vi "Configure Trigger.vi"   [LabVIEW 2015, in "LeCroy Wave Series.lvlib"]
doc: "This VI select the type of trigger."
uses:
  <instrlib>/LeCroy Wave Series/LeCroy Wave Series.lvlib
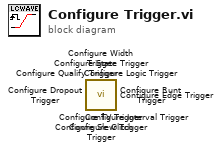
[diagram p0: block diagram]
diagram:
  n1 = call <instrlib>:"Configure TV Trigger.vi"() -> ()  [unwired: 14 in, 2 out]
  n2 = call <instrlib>:"Configure Logic Trigger.vi"() -> ()  [unwired: 14 in, 2 out]
  n3 = call <instrlib>:"Configure Dropout Trigger.vi"() -> ()  [unwired: 14 in, 2 out]
  n4 = call <instrlib>:"Configure Edge Trigger.vi"() -> ()  [unwired: 14 in, 2 out]
  n5 = call <instrlib>:"Configure Slew Trigger.vi"() -> ()  [unwired: 14 in, 2 out]
  n6 = call <instrlib>:"Configure State Trigger.vi"() -> ()  [unwired: 14 in, 2 out]
  n7 = call <instrlib>:"Configure Qualify Trigger.vi"() -> ()  [unwired: 14 in, 2 out]
  n8 = call <instrlib>:"Configure Interval Trigger.vi"() -> ()  [unwired: 14 in, 2 out]
  n9 = call <instrlib>:"Configure Runt Trigger.vi"() -> ()  [unwired: 14 in, 2 out]
  n10 = call <instrlib>:"Configure Glitch Trigger.vi"() -> ()  [unwired: 14 in, 2 out]
  n11 = call <instrlib>:"Configure Width Trigger.vi"() -> ()  [unwired: 14 in, 2 out]
